vi "Add Command.vi"(8 "error in":errorcluster, 11 "message refnum In":T1 format="%.0x") -> (0 "error out":errorcluster, 2 "command refnum":T1=18446744073709551615 format="%.0x", 3 "message refnum out":T1 format="%.0x")   [LabVIEW 2018, in "Instrument Addon Scripting API.lvlib"]
doc: "Adds or creates (if it does not already exists) a Command section to the specified Message. If the provided NodeID does not correspond to an existing Message section, this VI will throw an error."
uses:
  Instrument Addon Scripting API.lvlib
  <vilib>/NI Veristand/Custom Device API/Custom Device Item Ref.ctl
  <vilib>/NI Veristand/Custom Device API/Custom Device API.lvlib
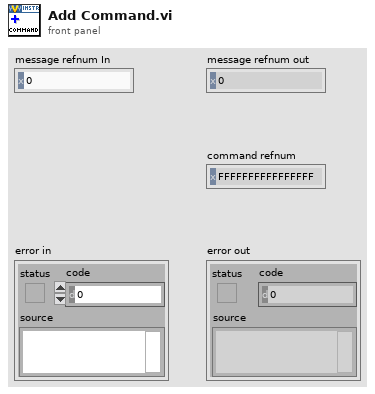
[diagram p1: front panel]
types:
  T1 = typedef "Custom Device API.lvlib/Custom Device Item Ref.ctl" = u64
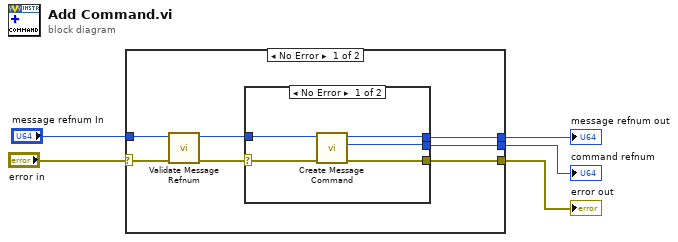
[diagram p0: block diagram]
diagram:
  n1 = case shown="No Error" "error in" {
    selector: "error in" -> [w8 w20]
    tunnel: "message refnum In" -> [w10 w21]
    tunnel: [w12 w21] -> w3
    tunnel: [w11 w20] -> w2
    tunnel: [w6 _] -> w1
    frame No Error {
      n2 = call "Validate Message Refnum.vi"("error in (no error)"=w8, "Message in"=w10) -> ("error out"=w7:errorcluster, "Message out"=w9:T1)  [unwired: 8 in]
      n3 = case shown="No Error" w7 {
        selector: w7 -> [w16 w18]
        tunnel: [w15 w19] -> w12
        tunnel: [w13 w18] -> w11
        tunnel: w9 -> [w17 w19]
        tunnel: [w14 _] -> w6
        frame No Error {
          n4 = call "Create Message Command.vi"("error in (no error)"=w16, "Message in"=w17) -> ("error out"=w13:errorcluster, "Command Section Ptr"=w14:T1, "Message out"=w15:T1)  [unwired: 7 in]
        }
        frame Error {
        }
      }
    }
    frame Error {
    }
  }
  "error out" <- w2
  "message refnum out" <- w3
  "command refnum" <- w1
